vi "StartStopAutomaticProgressBar.vi"(7 "Start / Stop ?":T1, 8 "error in (no error)":errorcluster) -> (0 "error out":errorcluster)   [LabVIEW 2011]
uses:
  Ctrls/EnumStartStopProgressBar.ctl
  030 - EVENTS/EnumFgvEventCommand.ctl
  030 - EVENTS/01 - ToHmiScheduler/ToHmiScheduler.ctl
  030 - EVENTS/01 - ToHmiScheduler/ToHmiSchedulerCommand.ctl
  030 - EVENTS/03 - ToMessageHandlerProcess/ToMessageHandlerEvent.ctl
  030 - EVENTS/03 - ToMessageHandlerProcess/enumMessageCriticity.ctl
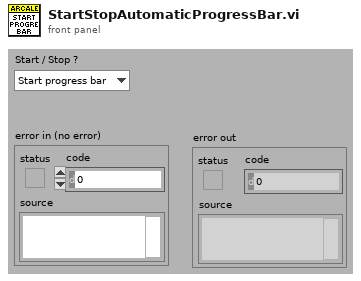
[diagram p1: front panel]
types:
  T1 = typedef "EnumStartStopProgressBar.ctl" = enum16{"Start progress bar", "Stop progress bar"}
  T2 = typedef "ToHmiSchedulerCommand.ctl" = enum16{"Load screen", "Lock screen", "Unlock screen", "Close enable", "Close disable", "Start automatic progress bar", "Stop automatic progress bar", "Set progress bar value (0..100)", "Load previous screen", "Close application", "View message", "Clear message", "Set Window State"}
  T3 = typedef "ToHmiScheduler.ctl" = cluster{"Command":T2, "Screen path":path, "Progress bar value":u8, "Screen Title":string, "To message handler event":T4, "Window_State":enum32{"Invalid", "Standard", "Closed", "Hidden", "Minimized", "Maximized"}}
  T4 = typedef "ToMessageHandlerEvent.ctl" = cluster{"date / time":timestamp, "Criticity":T5, "Emitter":string, "Message":string}
  T5 = typedef "enumMessageCriticity.ctl" = enum16{"No error", "Info", "Warning", "Error", "Fatal error"}
  T6 = typedef "EnumFgvEventCommand.ctl" = enum16{"Setup", "Cleanup", "Get"}
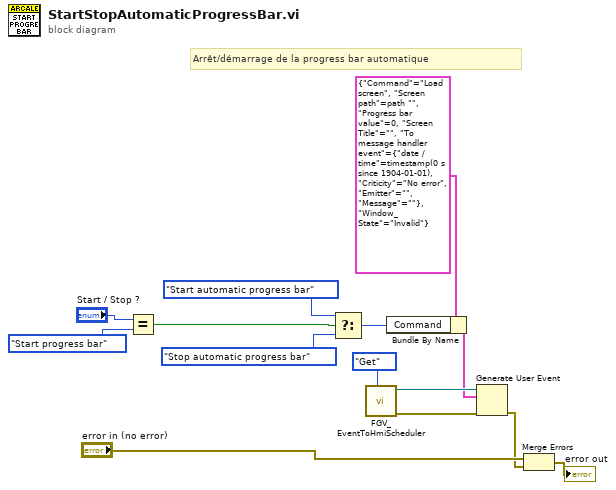
[diagram p0: block diagram]
diagram:
  # "Arrêt/démarrage de la progress bar automatique"
  n1 = Equal?(x="Start / Stop ?", y=EnumStartStopProgressBar."Start progress bar") -> (x = y?=w1:bool)
  n2 = Select(t=ToHmiSchedulerCommand."Start automatic progress bar" ("Command"), s=w1, f=ToHmiSchedulerCommand."Stop automatic progress bar" ("Command")) -> (s? t:f=w9:T2)
  n3 = call "FGV_EventToHmiScheduler.vi"("Command"=EnumFgvEventCommand."Get") -> ("error out"=w13:errorcluster, "ToHmiSchedulerEvent"=w12:refnum<user-event>)  [unwired: 9 in]
  n4 = Bundle By Name(cluster=T3 {"Command"=enum."Load screen", "Screen path"=path "", "Progress bar value"=0, "Screen Title"="", "To message handler event"={"date / time"=timestamp(0 s since 1904-01-01), "Criticity"=enum."No error", "Emitter"="", "Message"=""}, "Window_State"=enum."Invalid"} ("event data"), "Command"=w9) -> (w10:T3)
  n5 = Generate User Event(user event=w12, event data cluster=w10, error in=w13) -> (error out=w5:errorcluster)  [unwired: 1 out]
  n6 = Merge Errors("error in (no error)", w5) -> (→"error out":errorcluster)
